vi "Termék választás.vi"(8 "error in":errorcluster, 11 "Termék cluster array":T1[](array[typedef])) -> (0 "error out":errorcluster, 1 "Kiválasztott termék szám":i32, 2 "Kiválasztott termék":T1, 3 "OK":bool)   [LabVIEW 2014]
uses:
  <vilib>/Utility/miscctls.llb/LVRectTypeDef.ctl
  <vilib>/Utility/miscctls.llb/LVPointTypeDef.ctl
panel:
  in  "OK":bool
  in  "cancel":bool
  in  "Listbox":i32(listbox)
  # "Termék választás"
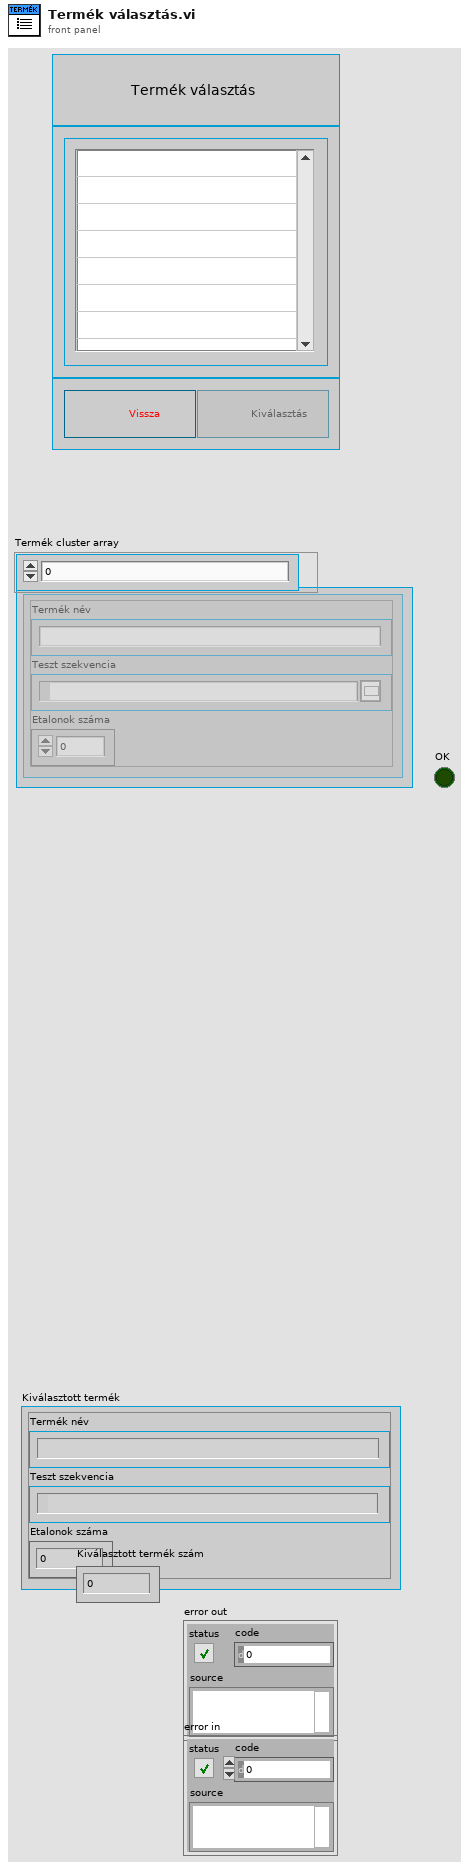
[diagram p1: front panel]
types:
  T1 = typedef "Termék cluster.ctl" = cluster{"Termék név":string, "Teszt szekvencia":path, "Etalonok száma":i8}
  T2 = typedef "LVPointTypeDef.ctl" = cluster{"Horizontal":i16, "Vertical":i16}
  T3 = typedef "LVRectTypeDef.ctl" = cluster{"Left":i16, "Top":i16, "Right":i16, "Bottom":i16}
  T4 = enum8{"Enabled", "Disabled", "Disabled and Grayed Out"}
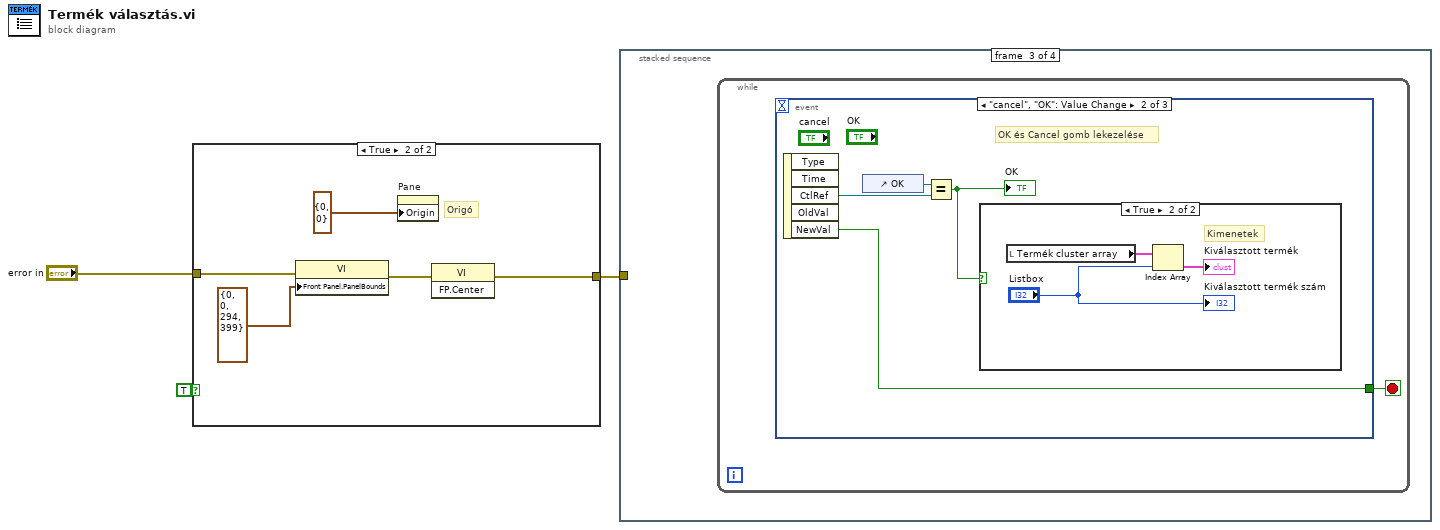
[diagram p0: block diagram]
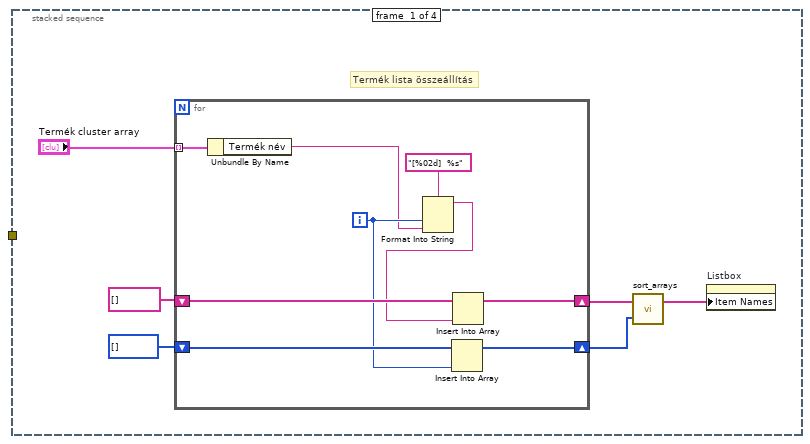
[diagram p3: hidden frame]
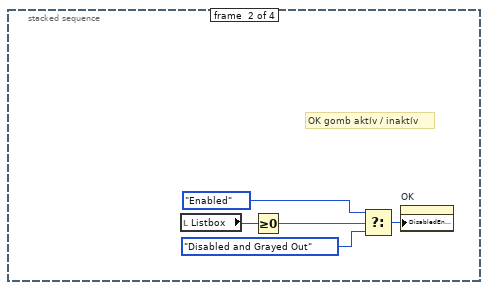
[diagram p4: hidden frame]
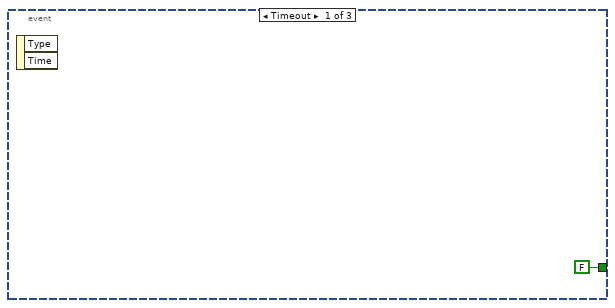
[diagram p5: hidden frame]
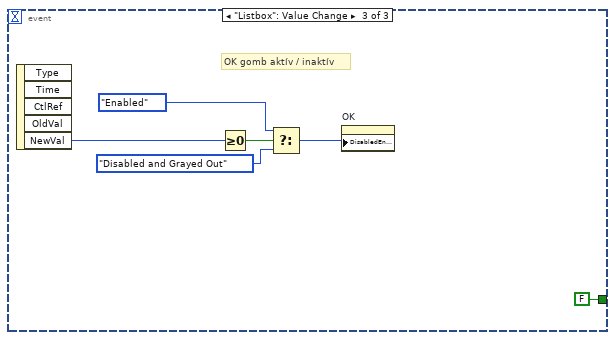
[diagram p7: hidden frame]
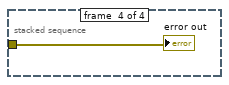
[diagram p8: hidden frame]
diagram:
  n1 = case shown="True" TRUE {
    tunnel: "error in" -> [w4 w7]
    tunnel: [w4 w5] -> w2
    frame False {
    }
    frame True {
      # "Origó"
      n2 = property class="VI"(error in=w7, "Front Panel.PanelBounds"=T3 {"Left"=0, "Top"=0, "Right"=294, "Bottom"=399} ("Front Panel Window:Panel Bounds")) -> (error out=w6:errorcluster)  [unwired: 1 in, 1 out]
      n3 = property on="Pane" class="Pane"("Origin"=T2 {"Horizontal"=0, "Vertical"=0}) -> ()  [unwired: 2 in, 2 out]
      n4 = invoke class="VI" method="FP.Center"(error in=w6) -> (error out=w5:errorcluster)  [unwired: 2 in, 2 out]
    }
  }
  n5 = stacked-sequence {
    tunnel: w2 -> [_ _ _ w45]
    frame #0 {
      # "Termék lista összeállítás"
      n6 = for {
        tunnel: "Termék cluster array" -> [w24] mode=indexing
        shift-right: [w22] -> w13
        shift-left: string[] [] ("Item Names") -> [w21]
        shift-right: [w19] -> w12
        shift-left: i32[] [] ("Indexes") -> [w20]
        i -> [w17]
        n7 = Unbundle By Name(w24) -> ("Termék név"=w16:string)
        n8 = Format Into String(format string="[%02d]  %s", w17, w16) -> (resulting string=w18:string)  [unwired: 2 in, 1 out]
        n9 = Insert Into Array(array=w20, new element=w17) -> (w19:i32[])  [unwired: 1 in]
        n10 = Insert Into Array(array=w21, new element=w18) -> (w22:string[])  [unwired: 1 in]
      }
      n11 = call "sort_arrays.vi"("index"=w12, "string"=w13) -> ("string 2"=w11:string[])  [unwired: 1 out]
      n12 = property on="Listbox" class="LstBox (strict)"("Item Names"=w11) -> ()  [unwired: 2 in, 2 out]
    }
    frame #1 {
      # "OK gomb aktív / inaktív"
      n13 = local read "Listbox"() -> (w29:i32)
      n14 = Greater Or Equal To 0?(x=w29) -> (x >= 0?=w25:bool)
      n15 = Select(t=T4."Enabled" ("Disabled"), s=w25, f=T4."Disabled and Grayed Out" ("Disabled")) -> (s? t:f=w26:T4)
      n16 = property on="OK" class="Bool"("DisabledEnum"=w26) -> ()  [unwired: 2 in, 2 out]
    }
    frame #2 {
      n17 = while {
        stop <- w30 stop-if-true
        n18 = event shown="[1] \"cancel\", \"OK\": Value Change" {
          selector: _ -> [_ _ _]
          dyn-events: _ -> [_ _ _]
          timeout: _ -> [_ _ _]
          tunnel: [FALSE ("NewVal") w35 FALSE ("NewVal")] -> w30
          event Timeout {
            n19 = event-data() -> ()  [unwired: 1 in, 2 out]
          }
          event "cancel", "OK": Value Change {
            # "OK és Cancel gomb lekezelése"
            n20 = event-data() -> ("CtlRef"=w33:refnum<vi>, "NewVal"=w35:bool)  [unwired: 1 in, 3 out]
            n21 = control-ref of="OK"() -> (w34:refnum<vi>)
            n22 = Equal?(x=w34, y=w33) -> (x = y?=w32:bool)
            "OK" <- w32
            n23 = case shown="True" w32 {
              frame False {
              }
              frame True {
                # "Kimenetek"
                n24 = local read "Termék cluster array"() -> (w37:T1[])
                n25 = Index Array(array=w37, index="Listbox") -> (element=→"Kiválasztott termék":T1)
                "Kiválasztott termék szám" <- "Listbox"
              }
            }
          }
          event "Listbox": Value Change {
            # "OK gomb aktív / inaktív"
            n26 = event-data() -> ("NewVal"=w44:i32)  [unwired: 1 in, 4 out]
            n27 = Greater Or Equal To 0?(x=w44) -> (x >= 0?=w43:bool)
            n28 = Select(t=T4."Enabled" ("Disabled"), s=w43, f=T4."Disabled and Grayed Out" ("Disabled")) -> (s? t:f=w40:T4)
            n29 = property on="OK" class="Bool"("DisabledEnum"=w40) -> ()  [unwired: 2 in, 2 out]
          }
        }
      }
    }
    frame #3 {
      "error out" <- w45
    }
  }
